vi "Log.CreateEventLog.vi"(4 "Base Log File Path":path, 6 "Array":T2[](array[typedef]), 7 "Sequence.AbortChannel":string, 8 "error in (no error)":errorcluster, 9 "Value":T4(ring), 10 "Station.ID":string, 11 ".NET Refnum in":T3) -> (0 "error out":errorcluster, 3 ".NET Refnum out":T1)   [LabVIEW 2015, in "Single Station Execution.lvlib"]
uses:
  Single Station Execution.lvlib
  <vilib>/NI Veristand/Execution/Workspace/WorkspaceAPI.ctl
  NationalInstruments.VeriStand.ClientAPI
  <vilib>/NI Veristand/Execution/DataLogging/TDMS Property.ctl
  <vilib>/NI Veristand/Execution/DataLogging/DataLoggingSpecification Ref.ctl
  <vilib>/NI Veristand/Execution/DataLogging/File Conflict Operation.ctl
  <vilib>/NI Veristand/Execution/DataLogging/Slope.ctl
  <vilib>/NI Veristand/Execution/DataLogging/New Data Logging Specification (TDMS).vi
  <vilib>/NI Veristand/Execution/DataLogging/Set Data Logging Rate (Target Rate).vi
  <vilib>/NI Veristand/Execution/DataLogging/Set Start Trigger (Digital Edge).vi
  <vilib>/NI Veristand/Execution/DataLogging/Set Stop Trigger (Duration).vi
  <vilib>/NI Veristand/Execution/DataLogging/NI_VS Data Logging API.lvlib
  <vilib>/NI Veristand/Execution/Workspace/NI_VS Workspace ExecutionAPI.lvlib
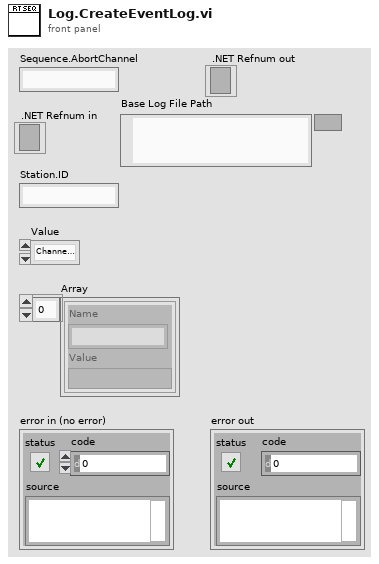
[diagram p1: front panel]
types:
  T1 = typedef "NI_VS Data Logging API.lvlib/DataLoggingSpecification Ref.ctl" = refnum<k24>
  T2 = typedef "NI_VS Data Logging API.lvlib/TDMS Property.ctl" = cluster{"Name":string, "Value":variant}
  T3 = typedef "NI_VS Workspace ExecutionAPI.lvlib/WorkspaceAPI.ctl" = refnum<k24>
  T4 = enum16{"Channels (No System Channel)", "Aliases", "All"}
  T5 = typedef "NI_VS Data Logging API.lvlib/Slope.ctl" = enum16{"Rising", "Falling"}
  T6 = typedef "NI_VS Data Logging API.lvlib/File Conflict Operation.ctl" = enum16{"Create Unique", "Append to Existing", "Overwrite"}
  T7 = typedef "NI_VS Data Logging API.lvlib/TDMS Channel Group.ctl" = cluster{"Group Name":string, "Group Description":string, "Group Properties":T2[], "Channels":T8[], "Time Channel Options":T9, "Time Channel Name":string}
  T8 = typedef "NI_VS Data Logging API.lvlib/TDMS Channel.ctl" = cluster{"Channel Name":string, "Channel Path":string, "Channel Description":string, "Channel Properties":T2[]}
  T9 = typedef "NI_VS Data Logging API.lvlib/Time Channel Options.ctl" = enum16{"No Time Channel", "Absolute Time", "System Time", "System Time - Microseconds", "Absolute Time as Double"}
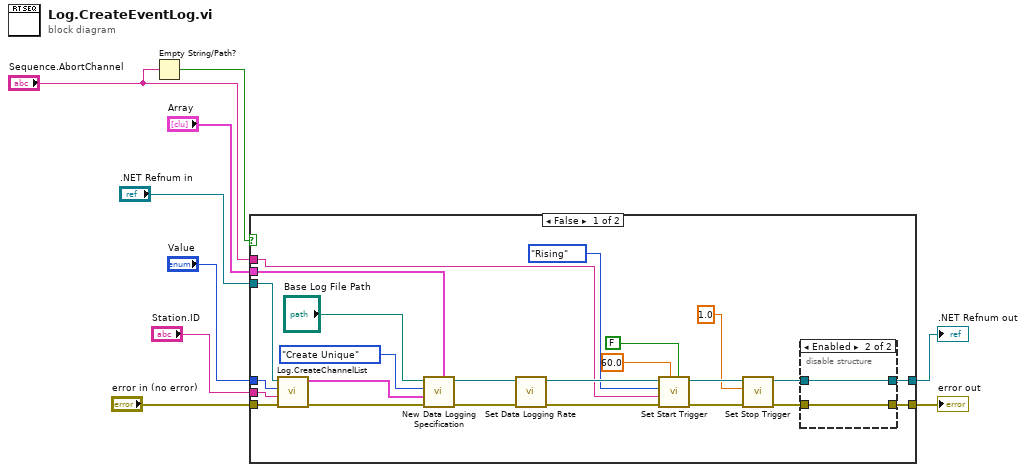
[diagram p0: block diagram]
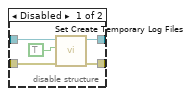
[diagram p2: hidden frame]
diagram:
  n1 = Empty String/Path?(string/path="Sequence.AbortChannel") -> (empty?=w1:bool)
  n2 = case shown="False" w1 {
    tunnel: "error in (no error)" -> [w33 w41]
    tunnel: [w12 w41] -> w3
    tunnel: "Sequence.AbortChannel" -> [w26 _]
    tunnel: [w11 _] -> w5
    tunnel: "Array" -> [w21 _]
    tunnel: ".NET Refnum in" -> [w15 _]
    tunnel: "Value" -> [w14 _]
    tunnel: "Station.ID" -> [w13 _]
    frame False {
      n3 = call "Log.CreateChannelList.vi"("error in (no error)"=w33, "Station.ID"=w13, "Value"=w14, "Workspace"=w15) -> ("error out"=w27:errorcluster, "Channel List"=w22:T7[])  [unwired: 6 in]
      n4 = call-poly <vilib>:"New Data Logging Specification.vi"("File Properties"=w21, "error in (no error)"=w27, "Channel Groups"=w22, "File Conflict Operation"=File_Conflict_Operation."Create Unique", "Base Log File Path"="Base Log File Path") -> ("error out"=w31:errorcluster, "Data Logging Specification Ref out"=w28:T1)  [unwired: 5 in]
      n5 = call-poly <vilib>:"Set Data Logging Rate.vi"("error in (no error)"=w31, "Data Logging Specification Ref in"=w28) -> ("error out"=w30:errorcluster, "Data Logging Specification Ref out"=w29:T1)  [unwired: 8 in]
      n6 = call-poly <vilib>:"Set Start Trigger.vi"("Retriggerable (F)"=FALSE, "Pre-Trigger Duration (0 s)"=60.0, "error in (no error)"=w30, "Trigger Channel"=w26, "Slope"=Slope."Rising", "Data Logging Specification Ref in"=w29) -> ("error out"=w20:errorcluster, "Data Logging Specification Ref out"=w17:T1)  [unwired: 4 in]
      n7 = call-poly <vilib>:"Set Stop Trigger.vi"("error in (no error)"=w20, "Duration"=1.0, "Data Logging Specification Ref in"=w17) -> ("error out"=w19:errorcluster, "Data Logging Specification Ref out"=w18:T1)  [unwired: 7 in]
      n8 = disable-structure shown="Enabled" {
        disable-tunnel: [w38 w39] -> w11
        disable-tunnel: [w37 w40] -> w12
        disable-tunnel: w19 -> [w35 w40]
        disable-tunnel: w18 -> [w34 w39]
        frame Disabled {
          n9 = call <vilib>:"Set Create Temporary Log Files.vi"("error in (no error)"=w35, "CreateTemporaryLogFiles"=TRUE, "Data Logging Specification Ref in"=w34) -> ("error out"=w37:errorcluster, "Data Logging Specification Ref out"=w38:T1)  [unwired: 7 in]
        }
        frame Enabled {
        }
      }
    }
    frame True {
    }
  }
  ".NET Refnum out" <- w5
  "error out" <- w3
